vi "Save Report SubVI.vi"(3 "File Name":string, 8 "error in (no error)":errorcluster, 9 "Fields":string[](array[string]), 10 "Inputs":string[](array[string]), 11 "Results File Location:":path) -> (0 "error out":errorcluster)   [LabVIEW 2018]
uses:
  <vilib>/Utility/NIReport.llb/Append Text Table to Report (wrap).vi
  <vilib>/Utility/NIReport.llb/NI_report.lvclass
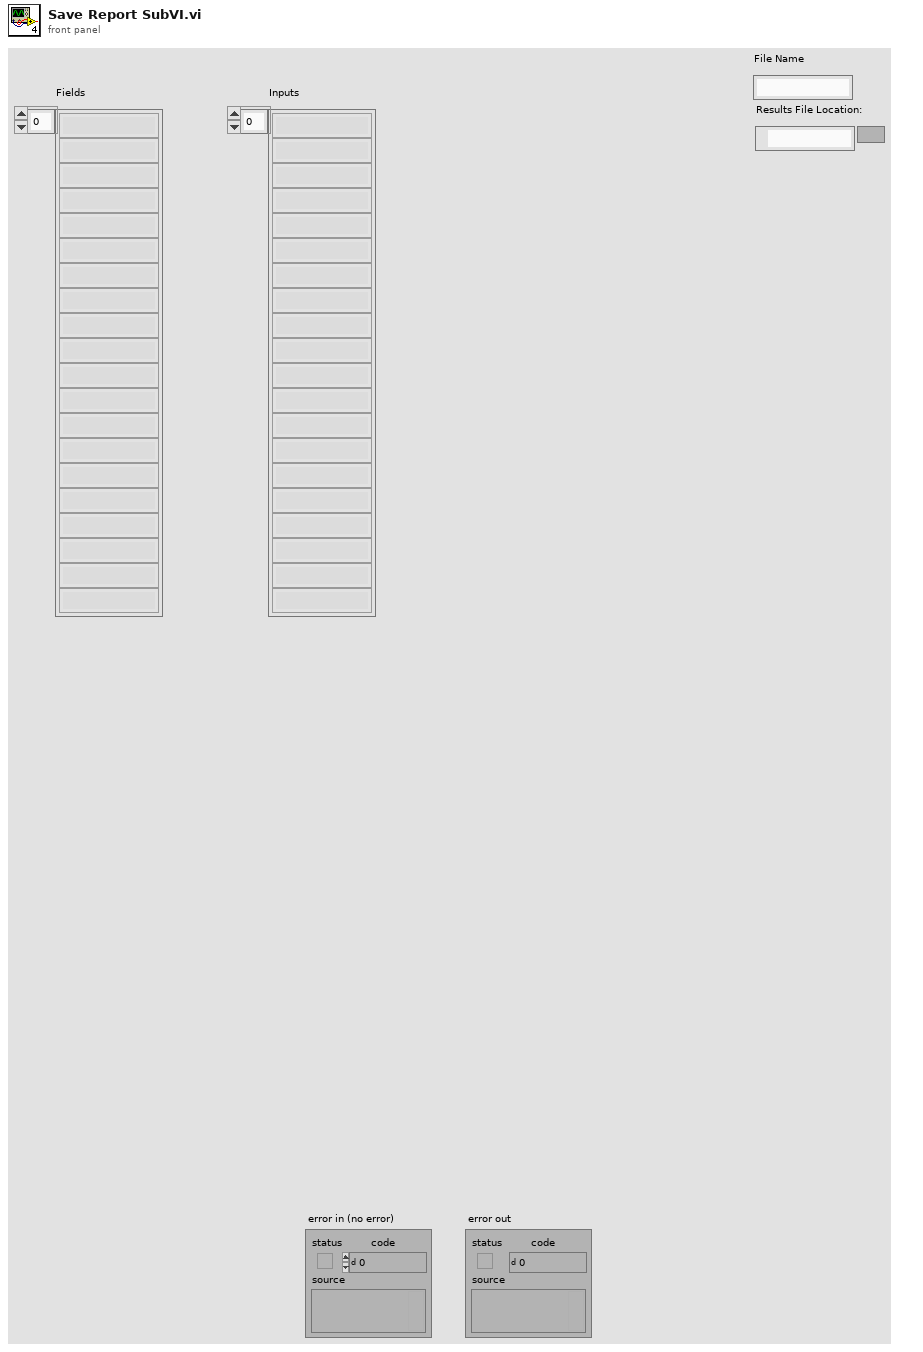
[diagram p1: front panel]
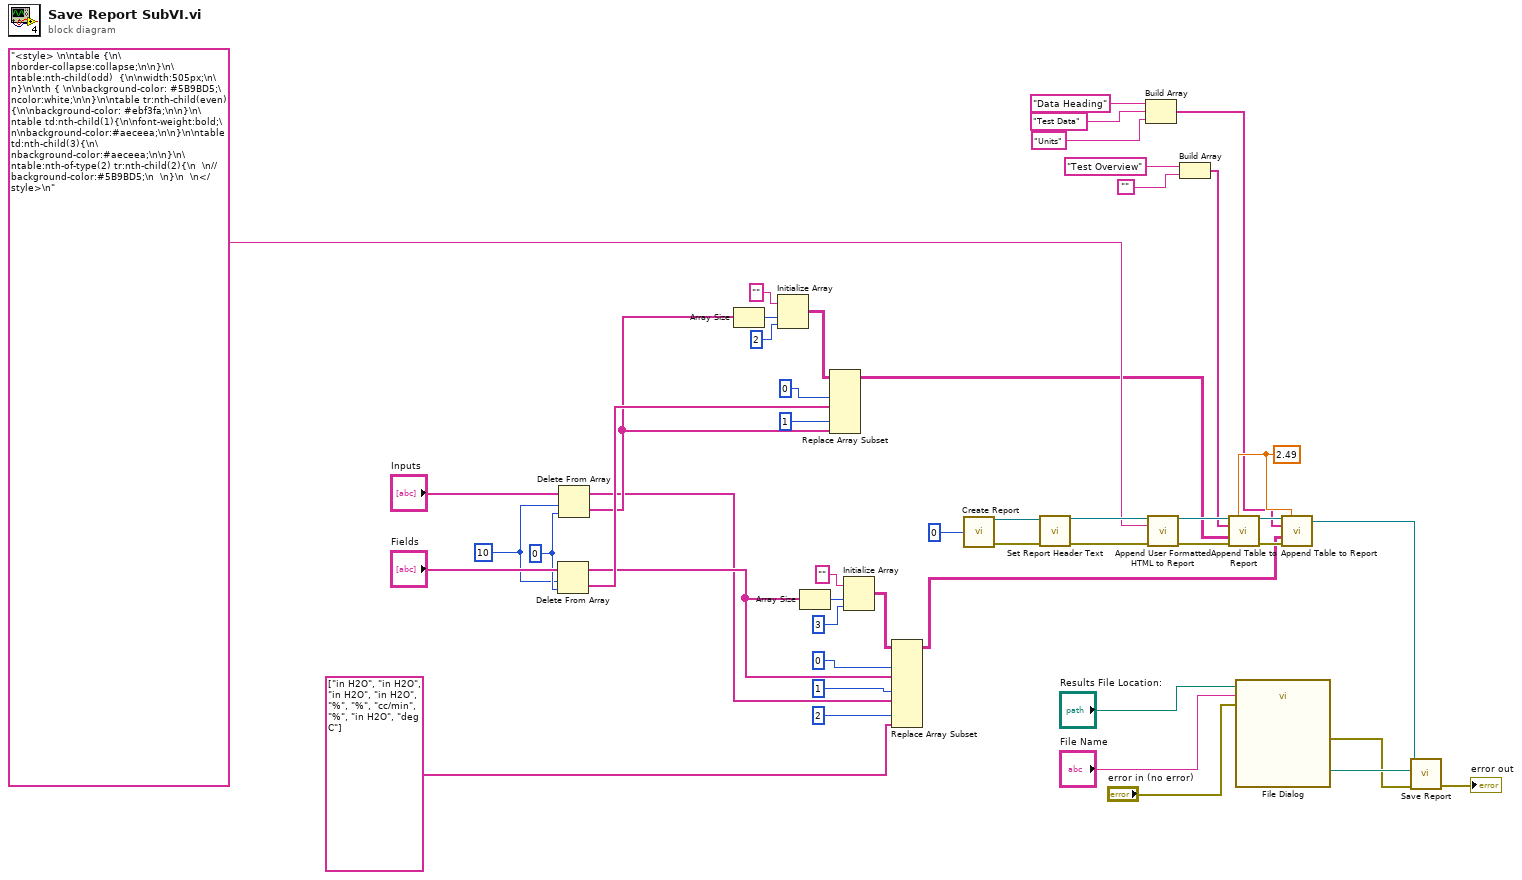
[diagram p0: block diagram]
diagram:
  w4 = 10 ("length")
  w5 = 0 ("index")
  w27 = 2.49
  n1 = Delete From Array(array="Fields", length=w4, index=w5) -> (deleted portion=w8:string[], array with subset deleted=w3:string[])
  n2 = Delete From Array(array="Inputs", length=w4, index=w5) -> (deleted portion=w6:string[], array with subset deleted=w2:string[])
  n3 = Array Size(array=w6) -> (size(s)=w40:i32)
  n4 = Initialize Array("", w40, 2 ("dimension size")) -> (w23:string[][])
  n5 = Array Size(array=w3) -> (size(s)=w18:i32)
  n6 = Replace Array Subset(array=w23, new element #1=w8, index (col) #1=0, new element #2=w6, index (col) #2=1) -> (w24:string[][])  [unwired: 2 in]
  n7 = Initialize Array("", w18, 3 ("dimension size")) -> (w16:string[][])
  n8 = Replace Array Subset(array=w16, new element #1=w3, index (col) #1=0, new element #2=w2, index (col) #2=1, new element #3=string[] ["in H2O", "in H2O", "in H2O", "in H2O", "%", "%", "cc/min", "%", "in H2O", "deg C"] ("Units"), index (col) #3=2) -> (w11:string[][])  [unwired: 3 in]
  n9 = call <vilib>:"Create Report.vi"("report type"=0) -> ("report out"=w37:refnum<class "NI_report.lvclass">, "error out"=w36:errorcluster)  [unwired: 13 in]
  n10 = call-dynamic "Set Report Header Text.vi"("report in"=w37, "error in (no error)"=w36) -> ("report out"=w34:refnum<class "NI_report.lvclass">, "error out"=w35:errorcluster)  [unwired: 12 in]
  n11 = Build Array("Data Heading", "Test Data", "Units") -> (w10:string[])
  n12 = call-dynamic "Append User Formatted HTML to Report.vi"("report in"=w34, "HTML text"="<style> \n\ntable {\n\nborder-collapse:collapse;\n\n}\n\ntable:nth-child(odd)  {\n\nwidth:505px;\n\n}\n\nth { \n\nbackground-color: #5B9BD5;\ncolor:white;\n\n}\n\ntable tr:nth-child(even) {\n\nbackground-color: #ebf3fa;\n\n}\n\ntable td:nth-child(1){\n\nfont-weight:bold;\n\nbackground-color:#aeceea;\n\n}\n\ntable td:nth-child(3){\n\nbackground-color:#aeceea;\n\n}\n\ntable:nth-of-type(2) tr:nth-child(2){\n  \n//background-color:#5B9BD5;\n  \n}\n  \n</style>\n", "error in (no error)"=w35) -> ("report out"=w33:refnum<class "NI_report.lvclass">, "error out"=w32:errorcluster)  [unwired: 11 in]
  n13 = Build Array("Test Overview", "") -> (w25:string[])
  n14 = call-poly <vilib>:"Append Table to Report.vi"("report in"=w33, "column width (1)"=w27, "column headers"=w25, "text data"=w24, "error in (no error)"=w32) -> ("report out"=w29:refnum<class "NI_report.lvclass">, "error out"=w28:errorcluster)  [unwired: 7 in, 2 out]
  n15 = call "File Dialog"("start path"="Results File Location:", "default name"="File Name", "error in"="error in (no error)") -> ("selected path"=w48:path, "error out"=w38:errorcluster)  [unwired: 9 in, 2 out]
  n16 = call-poly <vilib>:"Append Table to Report.vi"("report in"=w29, "column width (1)"=w27, "column headers"=w10, "text data"=w11, "error in (no error)"=w28) -> ("report out"=w26:refnum<class "NI_report.lvclass">)  [unwired: 7 in, 3 out]
  n17 = call "Save Report.vi"("error in (no error)"=w38, "Results File Location:"=w48, "NI_report in"=w26) -> ("error out"=→"error out":errorcluster)  [unwired: 5 in, 3 out]
